vi "Testing Config.vi"() -> ()   [LabVIEW 2026]
uses:
  ConfigCluster.ctl
  Config Clusters/Channel Setup/(Main) Channel Setup.ctl
  Config Clusters/Channel Setup/Channel Interfaces.ctl
  Config Clusters/Channel Setup/Micropulse.ctl
  Config Clusters/Channel Setup/Gates.ctl
  Config Clusters/Scan Setup/(Main) Scan Setup.ctl
  Config Clusters/Scan Setup/Scan Information.ctl
  Config Clusters/Scan Setup/Scan Settings.ctl
panel:
  out "cancelled 2":bool
  out "Bar ID":string
  out "Micropulse Voltage":dbl
  in  "Reset Btn":bool
  out "cancelled":bool
  in  "Path":path=path "D:/JOBS/27604 Tank 6 LabVIEW/TimetTankSixRepo/TimetTankSix/LabVIEW/Config/Test.txt"
  in  "Cluster 3":T1
  out "Cluster 2":T1
  in  "Load Button":bool
  in  "Save Button":bool
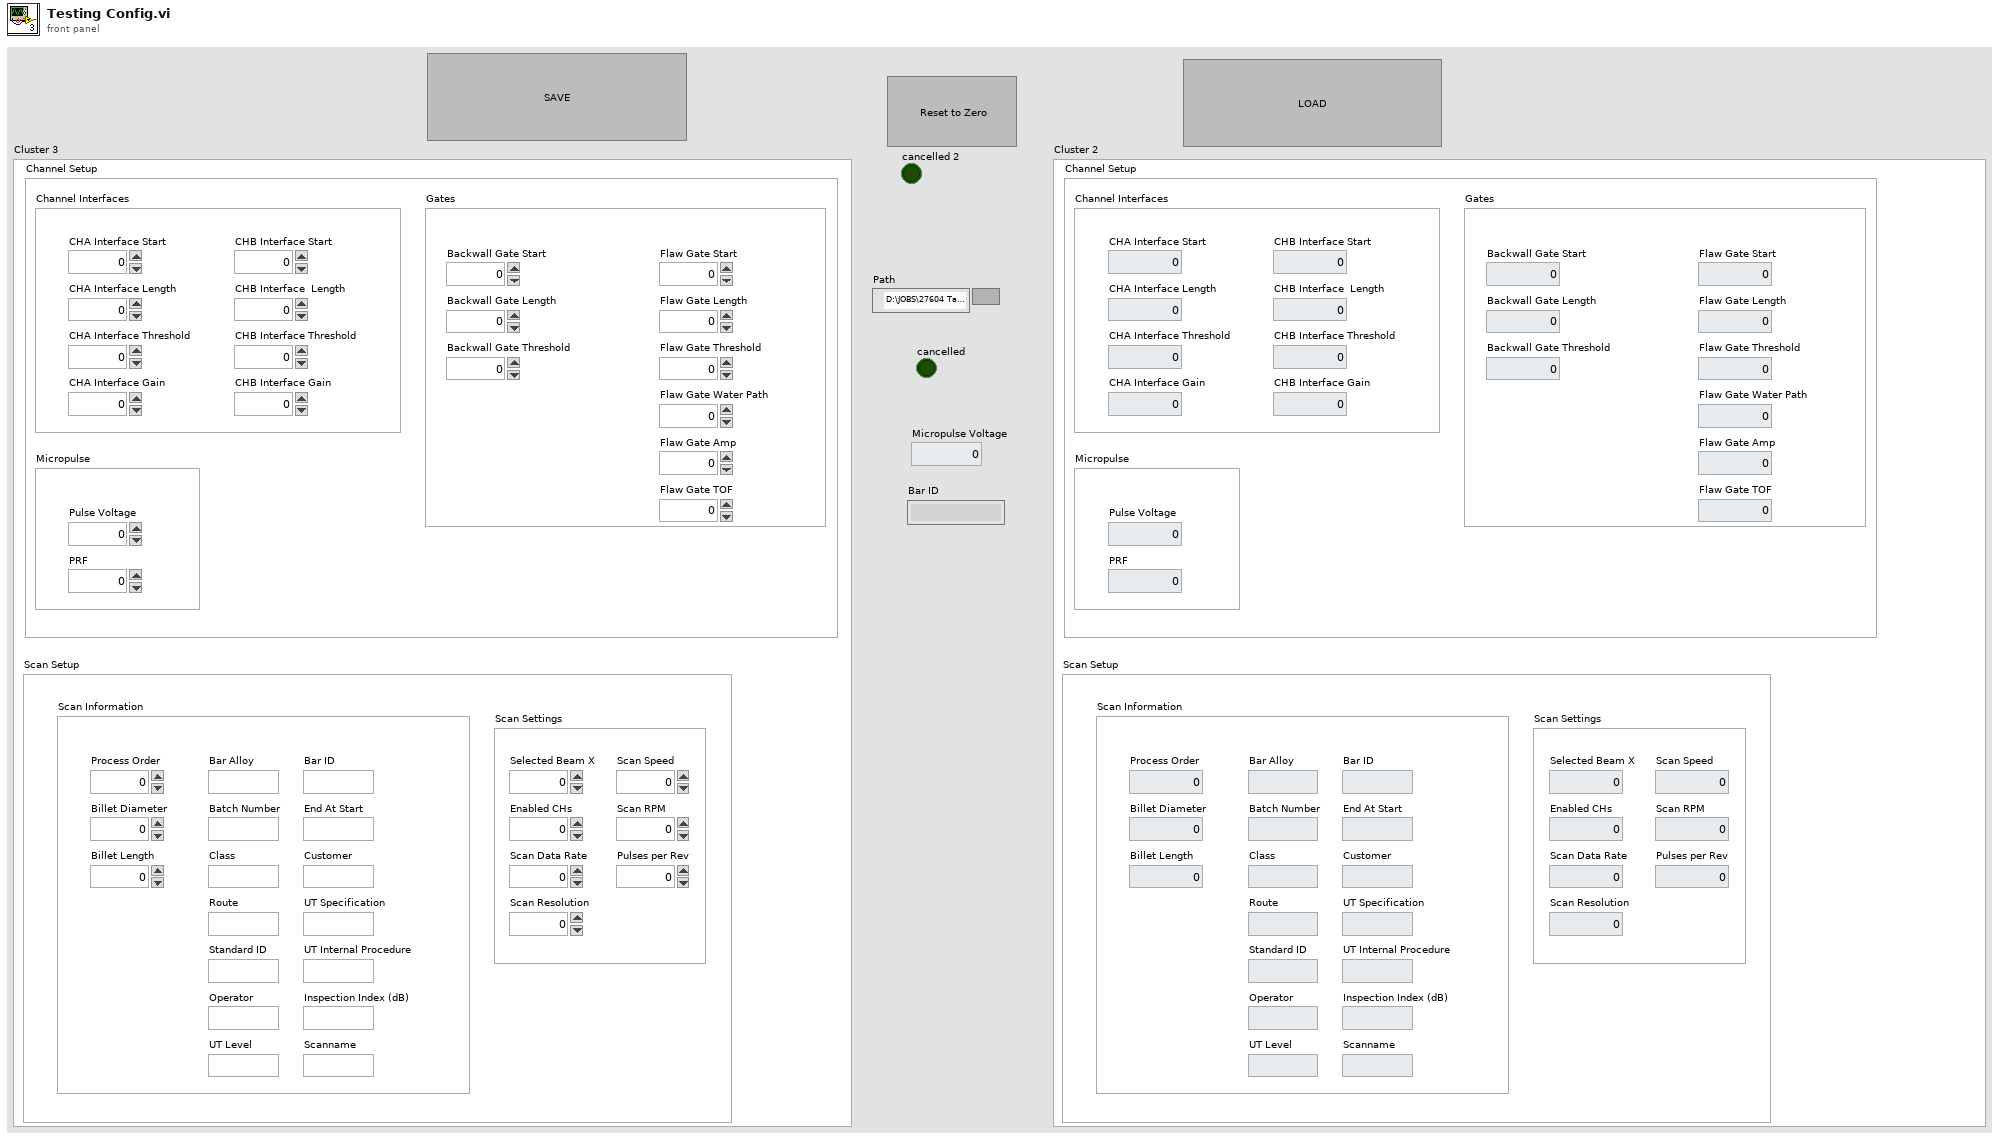
[diagram p1: front panel]
types:
  T1 = typedef "ConfigCluster.ctl" = cluster{"Channel Setup":T2, "Scan Setup":T6}
  T2 = typedef "(Main) Channel Setup.ctl" = cluster{"Channel Interfaces":T3, "Micropulse":T4, "Gates":T5}
  T3 = typedef "Channel Interfaces.ctl" = cluster{"CHA Interface Start":dbl, "CHA Interface Length":dbl, "CHA Interface Threshold":dbl, "CHA Interface Gain":dbl, "CHB Interface Start":dbl, "CHB Interface  Length ":dbl, "CHB Interface Threshold":dbl, "CHB Interface Gain":dbl}
  T4 = typedef "Micropulse.ctl" = cluster{"Pulse Voltage":dbl, "PRF":dbl}
  T5 = typedef "Gates.ctl" = cluster{"Backwall Gate Start":dbl, "Backwall Gate Length":dbl, "Backwall Gate Threshold":dbl, "Flaw Gate Start":dbl, "Flaw Gate Length":dbl, "Flaw Gate Threshold":dbl, "Flaw Gate Water Path":dbl, "Flaw Gate Amp":dbl, "Flaw Gate TOF":dbl}
  T6 = typedef "(Main) Scan Setup.ctl" = cluster{"Scan Information":T7, "Scan Settings":T8}
  T7 = typedef "Scan Information.ctl" = cluster{"Process Order":dbl, "Billet Diameter":dbl, "Billet Length":dbl, "Bar Alloy":string, "Batch Number":string, "Class":string, "Route":string, "Standard ID":string, "Bar ID":string, "End At Start":string, "Customer":string, "UT Specification":string, "UT Internal Procedure":string, "Operator":string, "UT Level":string, "Inspection Index (dB)":string, "Scanname":string}
  T8 = typedef "Scan Settings.ctl" = cluster{"Selected Beam X":dbl, "Enabled CHs":dbl, "Scan Data Rate":dbl, "Scan Resolution":dbl, "Scan Speed":dbl, "Scan RPM":dbl, "Pulses per Rev":dbl}
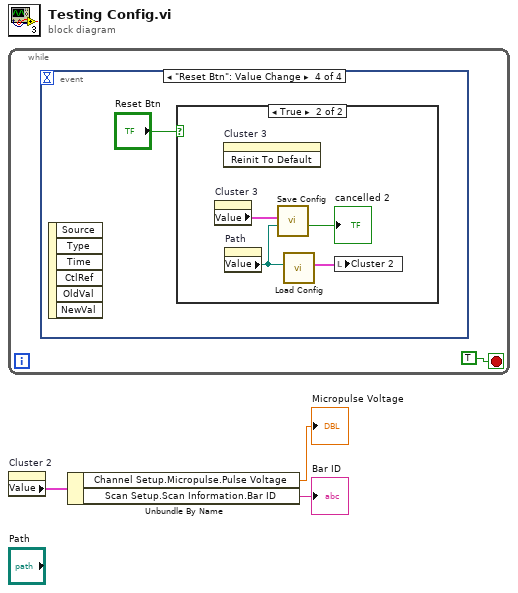
[diagram p0: block diagram]
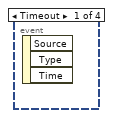
[diagram p2: hidden frame]
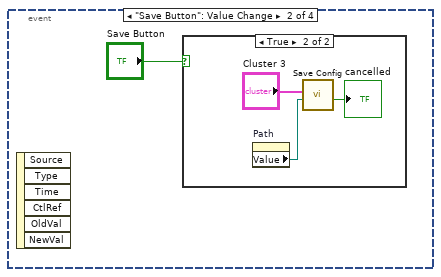
[diagram p3: hidden frame]
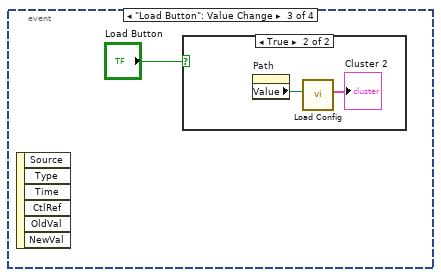
[diagram p5: hidden frame]
diagram:
  n1 = while {
    stop <- TRUE stop-if-true
    n2 = event shown="[3] \"Reset Btn\": Value Change" {
      selector: _ -> [_ _ _ _]
      dyn-events: _ -> [_ _ _ _]
      timeout: _ -> [_ _ _ _]
      event Timeout {
        n3 = event-data() -> ()  [unwired: 1 in, 3 out]
      }
      event "Save Button": Value Change {
        n4 = event-data() -> ()  [unwired: 1 in, 6 out]
        n5 = case shown="True" "Save Button" {
          frame False {
          }
          frame True {
            n6 = property on="Path" class="Path"() -> ("Value"=w6:path)  [unwired: 2 in, 2 out]
            n7 = call "Save Config.vi"("Path"=w6, "Cluster 2"="Cluster 3") -> ("cancelled"=→"cancelled":bool)  [unwired: 7 in, 2 out]
          }
        }
      }
      event "Load Button": Value Change {
        n8 = event-data() -> ()  [unwired: 1 in, 6 out]
        n9 = case shown="True" "Load Button" {
          frame False {
          }
          frame True {
            n10 = property on="Path" class="Path"() -> ("Value"=w11:path)  [unwired: 2 in, 2 out]
            n11 = call "Load Config.vi"("Path"=w11) -> ("Cluster 2"=→"Cluster 2":T1)  [unwired: 8 in, 1 out]
          }
        }
      }
      event "Reset Btn": Value Change {
        n12 = event-data() -> ()  [unwired: 1 in, 6 out]
        n13 = case shown="True" "Reset Btn" {
          frame False {
          }
          frame True {
            n14 = property on="Cluster 3" class="Clust (strict)"() -> ("Value"=w15:T1)  [unwired: 2 in, 2 out]
            n15 = invoke on="Cluster 3" class="Clust (strict)" method="Reinit To Default"() -> ()  [unwired: 3 in, 3 out]
            n16 = property on="Path" class="Path"() -> ("Value"=w13:path)  [unwired: 2 in, 2 out]
            n17 = call "Save Config.vi"("Path"=w13, "Cluster 2"=w15) -> ("cancelled"=→"cancelled 2":bool)  [unwired: 7 in, 2 out]
            n18 = call "Load Config.vi"("Path"=w13) -> ("Cluster 2"=w16:T1)  [unwired: 8 in, 1 out]
            n19 = local write "Cluster 2"(w16) -> ()
          }
        }
      }
    }
  }
  n20 = property on="Cluster 2" class="Clust (strict)"() -> ("Value"=w3:T1)  [unwired: 2 in, 2 out]
  n21 = Unbundle By Name(w3) -> ("Channel Setup.Micropulse.Pulse Voltage"=→"Micropulse Voltage":dbl, "Scan Setup.Scan Information.Bar ID"=→"Bar ID":string)
